vi "TBS读取波形2017.VI"() -> ()   [LabVIEW 2017]
uses:
  <vilib>/measure/matone.llb/Extract Single Tone Information 1 Chan.vi
  <vilib>/measure/NI_MAPro.lvlib
panel:
  in  "VISA资源名称":refnum<visa-resource-name>
  in  "要读的\n字节数":u32=1000 caption="所读字节数"
  out "幅值":dbl format="%.2p"
  out "YZEro":dbl
  out "单位":string
  out "YMUlt":dbl
  out "YOFf":dbl
  out "XZEro":dbl
  out "单位":string
  out "DeltX":dbl
  out "频率":dbl caption="波形频率" format="%.2p"
  out "波形图":waveform(dbl)(graph)
  # "读取示波器当前坐标轴信息"
  # "X轴"
  # "Y轴"
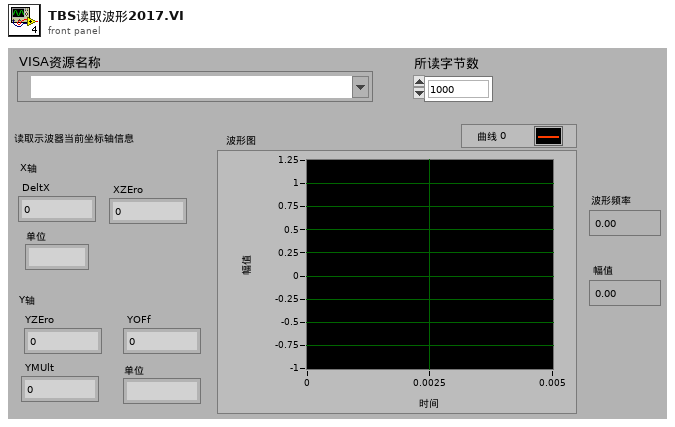
[diagram p1: front panel]
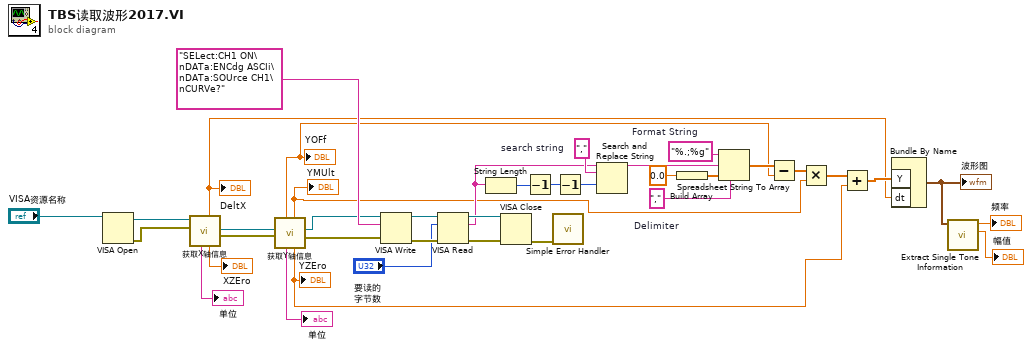
[diagram p0: block diagram]
diagram:
  w28 = ","  # search string
  w23 = ","  # Delimiter
  w31 = "%.;%g"  # Format String
  n1 = VISA Open(VISA resource name="VISA资源名称") -> (VISA resource name=w3:refnum<visa-resource-name>, error out=w2:errorcluster)  [unwired: 4 in]
  n2 = call "获取X轴信息.vi"("错误输入（无错误）"=w2, "VISA资源名称"=w3) -> ("错误输出"=w16:errorcluster, "VISA资源名称输出"=w17:refnum<visa-resource-name>, "XZEro"=→"XZEro":dbl, "DeltX"=w8:dbl, "XUNit"=→"单位":string)  [unwired: 3 in, 2 out]
  "DeltX" <- w8
  n3 = call "获取Y轴信息.vi"("错误输入（无错误）"=w16, "VISA资源名称"=w17) -> ("错误输出"=w14:errorcluster, "VISA资源名称输出"=w15:refnum<visa-resource-name>, "YZEro"=w5:dbl, "YMUlt"=w6:dbl, "YUNit"=→"单位":string, "YOFf"=w7:dbl)  [unwired: 4 in]
  "YOFf" <- w7
  "YMUlt" <- w6
  "YZEro" <- w5
  n4 = VISA Write(VISA resource name=w15, write buffer="SELect:CH1 ON\nDATa:ENCdg ASCIi\nDATa:SOUrce CH1\nCURVe?" ("string to write"), error in (no error)=w14) -> (VISA resource name out=w37:refnum<visa-resource-name>, error out=w36:errorcluster)  [unwired: 1 out]
  n5 = VISA Read(VISA resource name=w37, byte count="要读的\n字节数", error in (no error)=w36) -> (VISA resource name out=w35:refnum<visa-resource-name>, read buffer=w22:string, error out=w34:errorcluster)  [unwired: 1 out]
  n6 = String Length(string=w22) -> (length=w24:i32)
  n7 = VISA Close(VISA resource name=w35, error in (no error)=w34) -> (error out=w38:errorcluster)
  n8 = Decrement(x=w24) -> (x-1=w25:i32)
  n9 = call <vilib>:"Simple Error Handler.vi"("error in (no error)"=w38) -> ()  [unwired: 4 in, 5 out]
  n10 = Decrement(x=w25) -> (x-1=w26:i32)
  n11 = Search and Replace String(input string=w22, search string=w28, offset=w26) -> (result string=w27:string)  [unwired: 5 in, 3 out]
  n12 = Build Array(0.0) -> (w29:dbl[])
  n13 = Spreadsheet String To Array(delimiter (Tab)=w23, format string=w31, spreadsheet string=w27, array type (2D Dbl)=w29) -> (array=w21:dbl[])
  n14 = Subtract(x=w21, y=w7) -> (x-y=w20:dbl[])
  n15 = Multiply(x=w20, y=w6) -> (x*y=w9:dbl[])
  n16 = Add(x=w9, y=w5) -> (x+y=w10:dbl[])
  n17 = Bundle By Name("Y"=w10, "dt"=w8) -> (w19:waveform(dbl))  [unwired: 1 in]
  "波形图" <- w19
  n18 = call-poly <vilib>:"Extract Single Tone Information.vi"("time signal in"=w19) -> ("detected amplitude"=→"幅值":dbl, "detected frequency"=→"频率":dbl)  [unwired: 5 in, 4 out]
